vi "Enter_Temp_Press.vi"() -> ()   [LabVIEW 2013]
uses:
  Sub VIs/ADAM Controls/Ch_description_ADAM.ctl
  Sub VIs/ADAM Controls/Module_type_ADAM.ctl
  Sub VIs/ADAM Controls/Function_ADAM.ctl
  Sub VIs/ADAM Controls/Channel_State.ctl
  Sub VIs/ADAM Controls/Calib_type_ADAM.ctl
  Sub VIs/ADAM Controls/Address.ctl
  Anemometry/Anemometry Sub Vis/File/Setup_Filetype.ctl
  Sub VIs/ADAM Controls/Channel_names.ctl
  Anemometry/Anemometry Sub Vis/Controls/Preference_Mode.ctl
  Sub VIs/ADAM Controls/Update_scan_value.ctl
  Anemometry/Anemometry Sub Vis/Globals/Preference_global.vi
  Anemometry/Anemometry Sub Vis/Globals/Constants_global.vi
panel:
  in  "OK":bool
  out "Ch Description Array":T1[](array[typedef]) {"Duty" format="%.0b"; "D" format="%#_5g"; "C" format="%#_5g"; "B" format="%#_5g"; "A" format="%#_5g"}
  in  "mbars":dbl format="%#.1f"
  in  "Deg C":dbl format="%#.1f"
  in  "type specifier VI Refnum (for type only)":refnum<vi>
  out "Preference file":path
  in  "Server Comms":T7(ring)
  in  "Browse for Atmos Press":bool
  in  "Browse for Temp Ch":bool
  in  "Flow Pressure (Absolute) (mbars)":string="Froude:NPL:Atmos_Press"
  in  "Flow Temperature (deg C)":string="EnFlo Tun:Inlet Heater:Av Temp"
  # "DATA SOURCE"
  # "CURRENT VALUES"
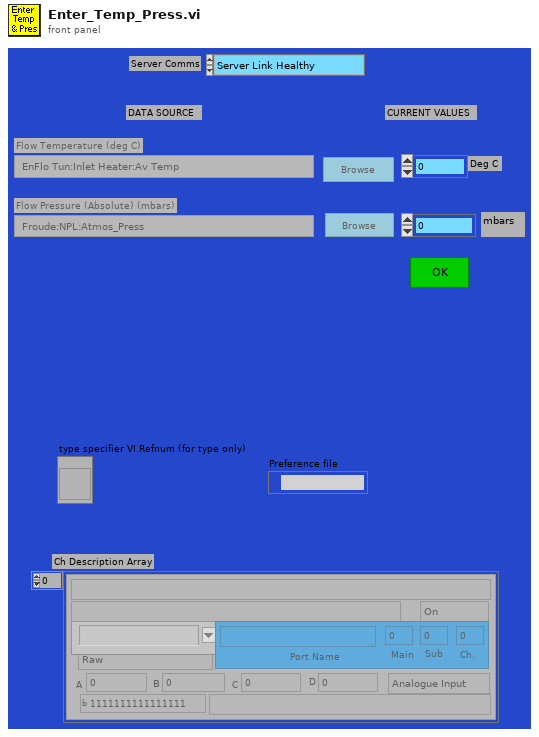
[diagram p1: front panel]
types:
  T1 = typedef "Ch_description_ADAM.ctl" = cluster{"Ch Name":string, "Type":T2, "Function":T3, "Ch State":T4, "Calibration type":T5, "A":dbl, "B":dbl, "C":dbl, "D":dbl, "Comments":string, "Address":T6, "String":string, "Duty":u16}
  T2 = typedef "Module_type_ADAM.ctl" = string
  T3 = typedef "Function_ADAM.ctl" = enum16{"Analogue Input", "Digital Input", "Event counter", "Event rate", "Analogue Output", "Digital Output", "Relay Output"}
  T4 = typedef "Channel_State.ctl" = enum16{"On", "Off", "Always On", "Always Off"}
  T5 = typedef "Calib_type_ADAM.ctl" = enum16{"Raw", "Bx + A", "Cx^2 + Bx + A", "Dx^3 + Cx^2 + Bx + A", "In Band", "Hi-Tec Q", "Hi-Tec M_dot", "Text"}
  T6 = typedef "Address.ctl" = cluster{"Main":i32, "Ch.":i32, "Sub":i32, "Port Name":string}
  T7 = enum16{"Server Link Healthy", "Do Not Link To Server"}
  T8 = typedef "Setup_Filetype.ctl" = enum16{"Measurement Setups", "Calibration Setups", "General", "Results File Plotter Setups", "Speed Calib Tweaks"}
  T9 = typedef "Channel_names.ctl" = enum16{"Active Only", "Active + Off", "All Channels"}
  T10 = enum16{"Zero or one", "One", "Zero or more", "One or more"}
  T11 = typedef "Preference_Mode.ctl" = enum16{"Load Preferences from file", "Save Preferences to file", "Load, Edit then Save"}
  T12 = typedef "Server_Comms.ctl" = enum16{"Server Link Healthy", "Do Not Link To Server"}
  T13 = typedef "Update_scan_value.ctl" = cluster{"Channel Name":string, "New Value":dbl}
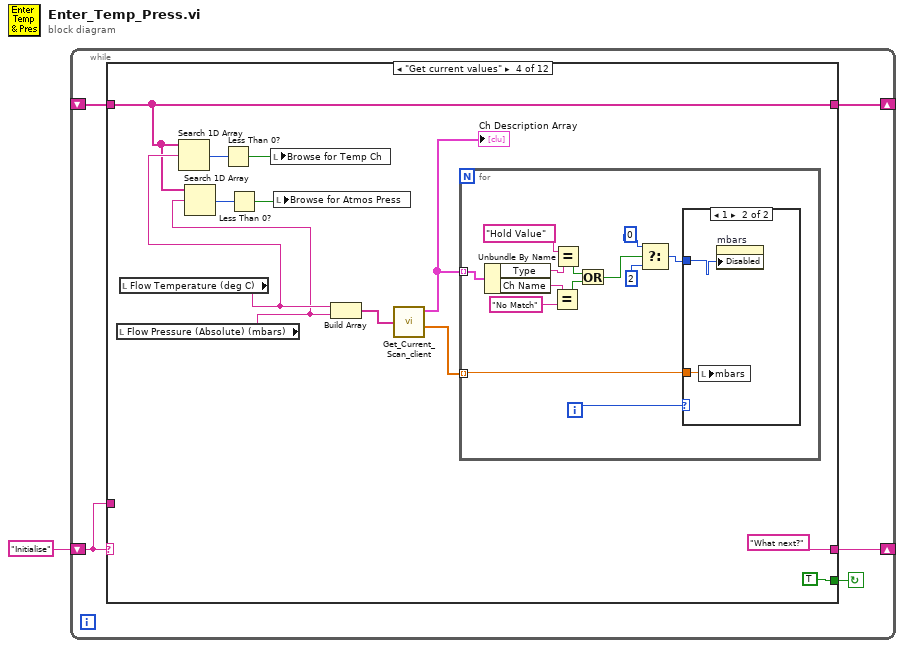
[diagram p0: block diagram]
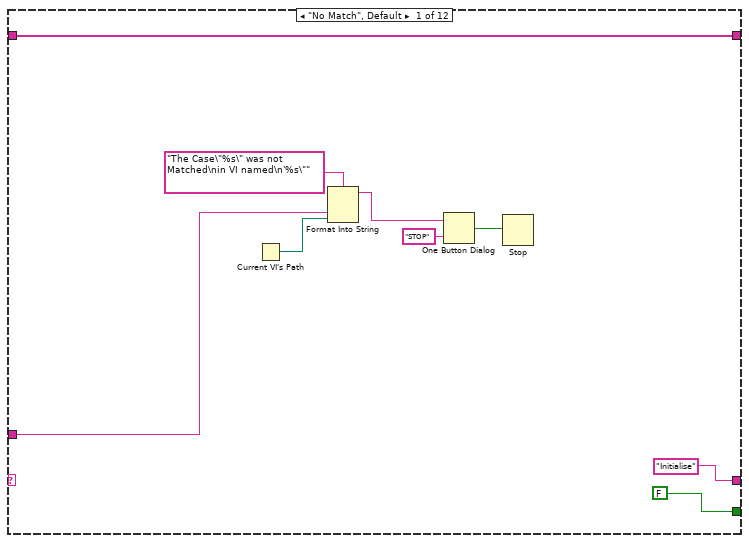
[diagram p2: hidden frame]
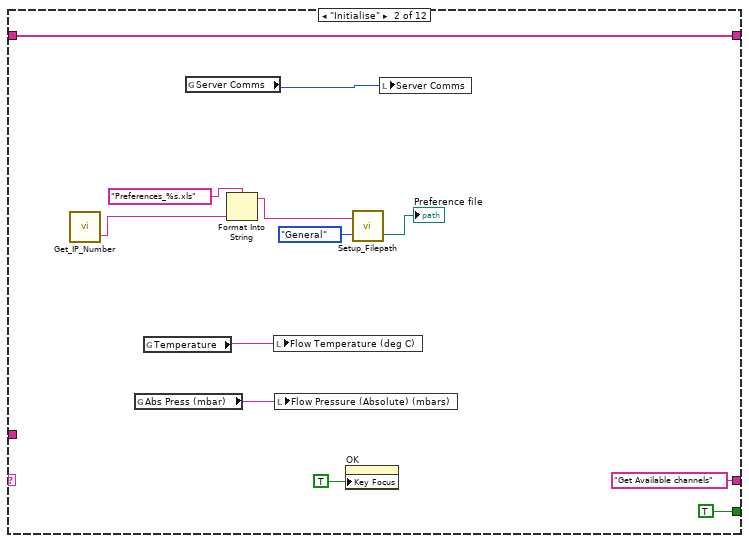
[diagram p3: hidden frame]
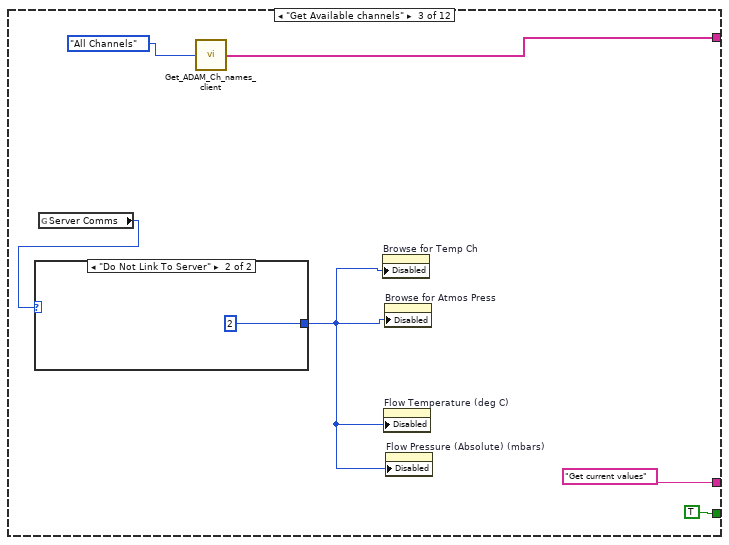
[diagram p4: hidden frame]
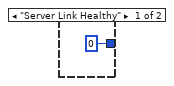
[diagram p5: hidden frame]
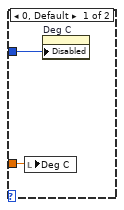
[diagram p6: hidden frame]
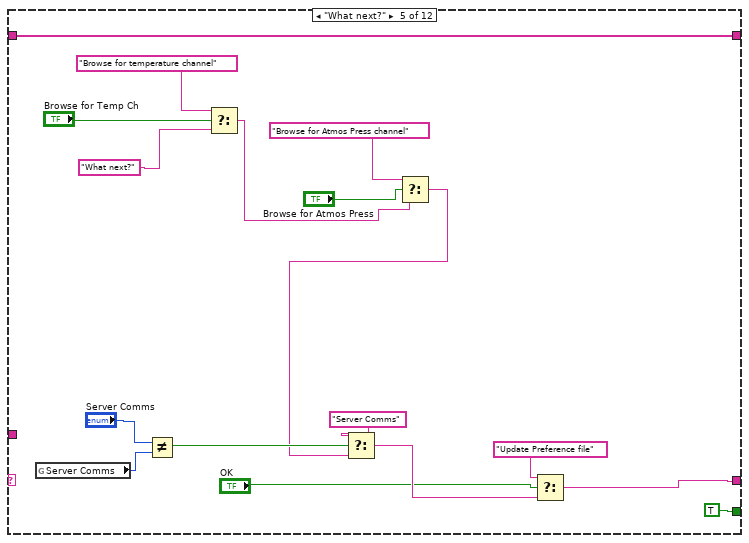
[diagram p7: hidden frame]
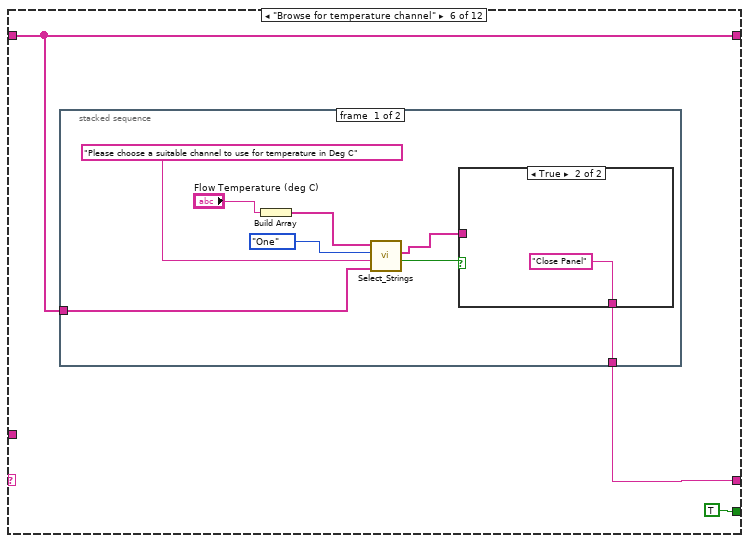
[diagram p8: hidden frame]
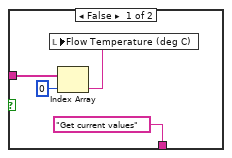
[diagram p9: hidden frame]
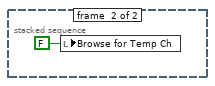
[diagram p10: hidden frame]
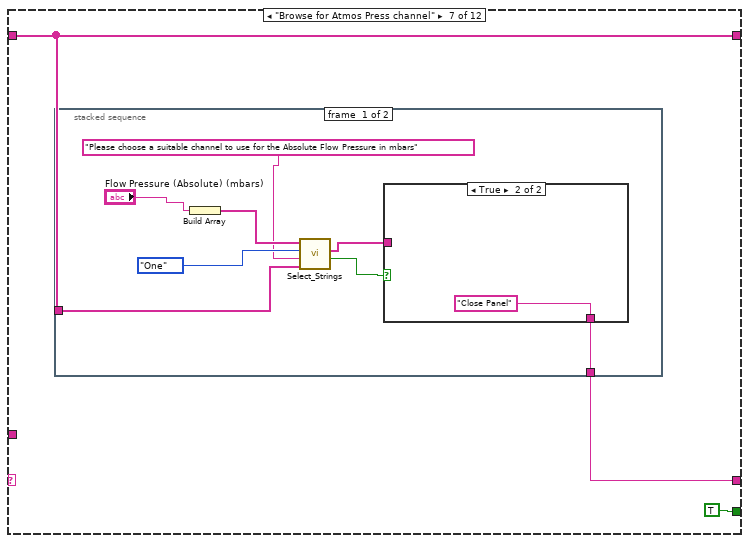
[diagram p11: hidden frame]
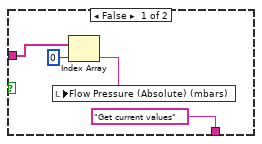
[diagram p12: hidden frame]
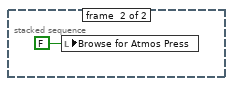
[diagram p13: hidden frame]
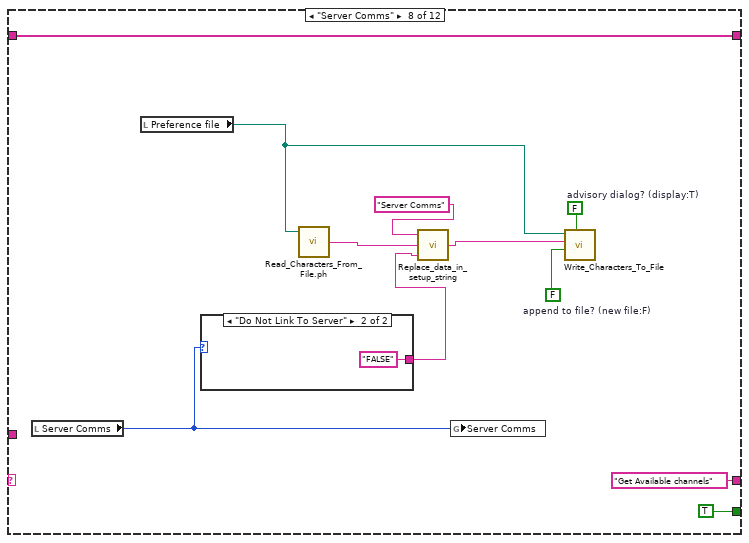
[diagram p14: hidden frame]
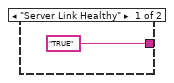
[diagram p15: hidden frame]
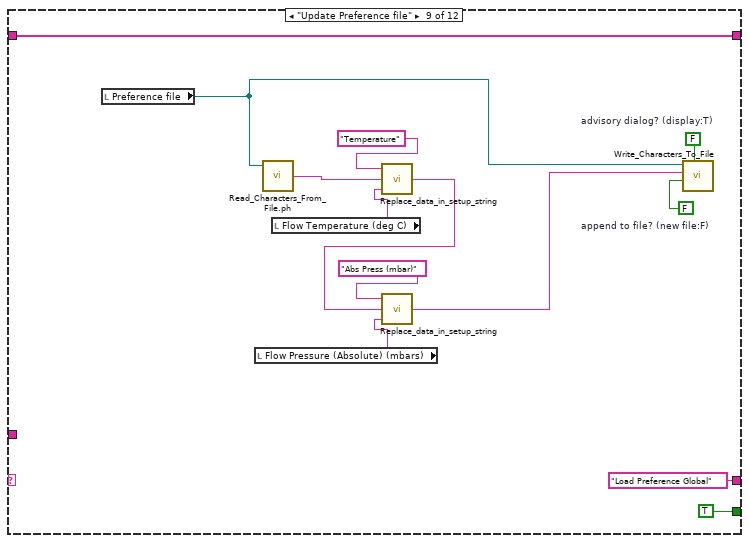
[diagram p16: hidden frame]
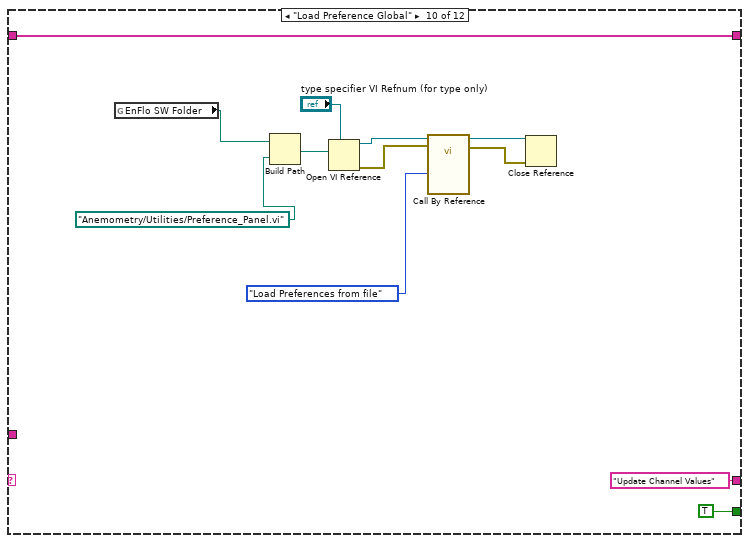
[diagram p17: hidden frame]
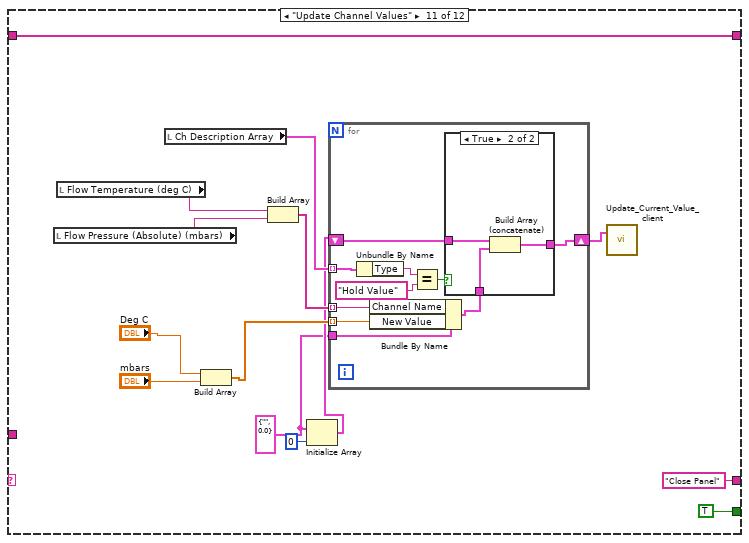
[diagram p18: hidden frame]
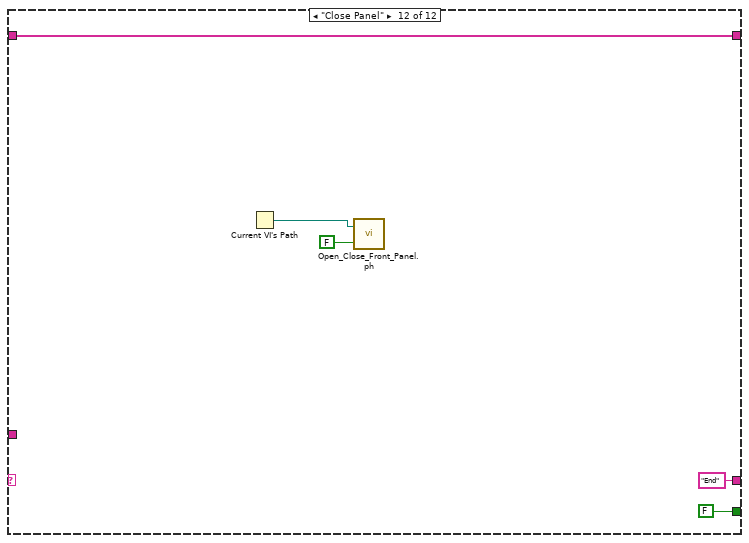
[diagram p20: hidden frame]
diagram:
  n1 = while {
    shift-left: "Initialise" -> [w4]
    shift-right: [w5] -> _
    shift-right: [w3] -> _
    shift-left: _ -> [w2]
    stop <- w6 continue-if-true
    n2 = case shown="\"Get current values\"" w4 {
      tunnel: [FALSE TRUE TRUE TRUE TRUE TRUE TRUE TRUE TRUE TRUE TRUE FALSE] -> w6
      tunnel: ["Initialise" "Get Available channels" "Get current values" "What next?" w78 w82 w99 "Get Available channels" "Load Preference Global" "Update Channel Values" "Close Panel" "End"] -> w5
      tunnel: w4 -> [w10 _ _ _ _ _ _ _ _ _ _ _]
      tunnel: [w7 w26 w30 w37 w75 w83 w100 w124 w139 w151 w165 w184] -> w3
      tunnel: w2 -> [w7 w26 _ w37 w75 w83 w100 w124 w139 w151 w165 w184]
      frame "No Match", Default {
        n3 = Current VI's Path() -> (path=w9:path)
        n4 = Format Into String(format string="The Case\"%s\" was not Matched\nin VI named\n'%s\"" ("Format String"), w10, w9) -> (resulting string=w13:string)  [unwired: 2 in, 1 out]
        n5 = One Button Dialog(message=w13, button name ("OK")="STOP") -> (true=w11:bool)
        n6 = Stop(stop? (T)=w11) -> ()
      }
      frame "Initialise" {
        n7 = call "Get_IP_Number.vi"() -> ("Computer Name"=w17:string)  [unwired: 1 out]
        n8 = global read "Preference_global.vi" "Abs Press (mbar)"() -> (w23:string)
        n9 = global read "Preference_global.vi" "Temperature"() -> (w22:string)
        n10 = global read "Preference_global.vi" "Server Comms"() -> (w27:T12)
        n11 = Format Into String(format string="Preferences_%s.xls" ("name or relative path"), w17) -> (resulting string=w18:string)  [unwired: 2 in, 1 out]
        n12 = local write "Flow Temperature (deg C)"(w22) -> ()
        n13 = local write "Flow Pressure (Absolute) (mbars)"(w23) -> ()
        n14 = property on="OK" class="Bool"("Key Focus"=TRUE) -> ()  [unwired: 2 in, 2 out]
        n15 = call "Setup_Filepath.vi"("Setup File Type"=Setup_Filetype."General", "Filename in"=w18) -> ("Filename Out"=→"Preference file":path)  [unwired: 1 out]
        n16 = local write "Server Comms"(w27) -> ()
      }
      frame "Get Available channels" {
        n17 = global read "Preference_global.vi" "Server Comms"() -> (w29:T12)
        n18 = case shown="\"Do Not Link To Server\"" w29 {
          tunnel: [u8 0 ("Disabled") u8 2 ("Disabled")] -> w28
          frame "Server Link Healthy" {
          }
          frame "Do Not Link To Server" {
          }
        }
        n19 = call "Get_ADAM_Ch_names_client.vi"("Channel names set"=Channel_names."All Channels") -> ("Ch names"=w30:string[])
        n20 = property on="Browse for Temp Ch" class="Bool (strict)"("Disabled"=w28) -> ()  [unwired: 2 in, 2 out]
        n21 = property on="Flow Temperature (deg C)" class="Str"("Disabled"=w28) -> ()  [unwired: 2 in, 2 out]
        n22 = property on="Browse for Atmos Press" class="Bool (strict)"("Disabled"=w28) -> ()  [unwired: 2 in, 2 out]
        n23 = property on="Flow Pressure (Absolute) (mbars)" class="Str"("Disabled"=w28) -> ()  [unwired: 2 in, 2 out]
      }
      frame "Get current values" {
        n24 = local read "Flow Pressure (Absolute) (mbars)"() -> (w36:string)
        n25 = local read "Flow Temperature (deg C)"() -> (w42:string)
        n26 = Search 1D Array(1D array=w37, element=w42) -> (index of element=w41:i32)  [unwired: 1 out]
        n27 = Search 1D Array(1D array=w37, element=w36) -> (index of element=w40:i32)  [unwired: 1 out]
        n28 = Less Than 0?(x=w41) -> (x < 0?=w39:bool)
        n29 = Less Than 0?(x=w40) -> (x < 0?=w38:bool)
        n30 = local write "Browse for Temp Ch"(w39) -> ()
        n31 = local write "Browse for Atmos Press"(w38) -> ()
        n32 = Build Array(w42, w36) -> (w45:string[])
        n33 = call "Get_Current_Scan_client.vi"("ADAM Ch Names"=w45) -> ("Ch Description Array"=w43:T1[], "Numerical Values"=w44:dbl[])  [unwired: 1 in, 1 out]
        "Ch Description Array" <- w43
        n34 = for {
          tunnel: w44 -> [w51] mode=indexing
          tunnel: w43 -> [w48] mode=indexing
          i -> [w60]
          n35 = Unbundle By Name(w48) -> ("Type"=w50:T2, "Ch Name"=w49:string)
          n36 = Equal?(x=w49, y="No Match") -> (x = y?=w54:bool)
          n37 = Equal?(x=T2 "Hold Value" ("Type"), y=w50) -> (x = y?=w53:bool)
          n38 = Or(x=w53, y=w54) -> (x .or. y?=w52:bool)
          n39 = Select(t=u8 0 ("Disabled"), s=w52, f=u8 2 ("Disabled")) -> (s? t:f=w56:u8)
          n40 = case shown="1" w60 {
            tunnel: w51 -> [w62 w64]
            tunnel: w56 -> [w61 w63]
            frame 0, Default {
              n41 = local write "Deg C"(w62) -> ()
              n42 = property on="Deg C" class="DigNum (strict)"("Disabled"=w61) -> ()  [unwired: 2 in, 2 out]
            }
            frame 1 {
              n43 = local write "mbars"(w64) -> ()
              n44 = property on="mbars" class="DigNum (strict)"("Disabled"=w63) -> ()  [unwired: 2 in, 2 out]
            }
          }
        }
      }
      frame "What next?" {
        n45 = global read "Preference_global.vi" "Server Comms"() -> (w69:T12)
        n46 = Not Equal?(x="Server Comms", y=w69) -> (x != y?=w67:bool)
        n47 = Select(t="Browse for temperature channel", s="Browse for Temp Ch", f="What next?") -> (s? t:f=w72:string)
        n48 = Select(t="Browse for Atmos Press channel", s="Browse for Atmos Press", f=w72) -> (s? t:f=w65:string)
        n49 = Select(t="Server Comms", s=w67, f=w65) -> (s? t:f=w71:string)
        n50 = Select(t="Update Preference file", s="OK", f=w71) -> (s? t:f=w78:string)
      }
      frame "Browse for temperature channel" {
        n51 = stacked-sequence {
          tunnel: w83 -> [w90 _]
          tunnel: [w85 _] -> w82
          frame #0 {
            n52 = Build Array("Flow Temperature (deg C)") -> (w92:string[])
            n53 = call "Select_Strings.vi"("Available Ch names"=w90, "Message"="Please choose a suitable channel to use for temperature in Deg C", "Selector mode"=T10."One", "Desired Ch names (in)"=w92) -> ("Cancel"=w86:bool, "Selected Channel Names"=w89:string[])  [unwired: 3 out]
            n54 = case shown="True" w86 {
              tunnel: w89 -> [w96 _]
              tunnel: ["Get current values" "Close Panel"] -> w85
              frame False {
                n55 = Index Array(array=w96, index=0) -> (element=w94:string)
                n56 = local write "Flow Temperature (deg C)"(w94) -> ()
              }
              frame True {
              }
            }
          }
          frame #1 {
            n57 = local write "Browse for Temp Ch"(FALSE ("Browse for Temp Ch")) -> ()
          }
        }
      }
      frame "Browse for Atmos Press channel" {
        n58 = stacked-sequence {
          tunnel: w100 -> [w107 _]
          tunnel: [w102 _] -> w99
          frame #0 {
            n59 = Build Array("Flow Pressure (Absolute) (mbars)") -> (w109:string[])
            n60 = call "Select_Strings.vi"("Available Ch names"=w107, "Message"="Please choose a suitable channel to use for the Absolute Flow Pressure in mbars", "Selector mode"=T10."One", "Desired Ch names (in)"=w109) -> ("Cancel"=w103:bool, "Selected Channel Names"=w106:string[])  [unwired: 3 out]
            n61 = case shown="True" w103 {
              tunnel: w106 -> [w113 _]
              tunnel: ["Get current values" "Close Panel"] -> w102
              frame False {
                n62 = Index Array(array=w113, index=0) -> (element=w111:string)
                n63 = local write "Flow Pressure (Absolute) (mbars)"(w111) -> ()
              }
              frame True {
              }
            }
          }
          frame #1 {
            n64 = local write "Browse for Atmos Press"(FALSE ("Browse for Atmos Press")) -> ()
          }
        }
      }
      frame "Server Comms" {
        w123 = FALSE  # append to file? (new file:F)
        w122 = FALSE  # advisory dialog? (display:T)
        n65 = local read "Server Comms"() -> (w117:T7)
        n66 = local read "Preference file"() -> (w119:path)
        n67 = case shown="\"Do Not Link To Server\"" w117 {
          tunnel: ["TRUE" "FALSE"] -> w116
          frame "Server Link Healthy" {
          }
          frame "Do Not Link To Server" {
          }
        }
        n68 = call "Read_Characters_From_File.ph.vi"("file path (dialog if empty)"=w119) -> ("character string"=w121:string)  [unwired: 1 in, 7 out]
        n69 = call "Replace_data_in_setup_string.vi"("New data string"=w116, "Input string"=w121, "Variable name"="Server Comms") -> ("Appended string"=w120:string)
        n70 = global write "Preference_global.vi" "Server Comms"(w117) -> ()
        n71 = call "Write_Characters_To_File.vi"("file path (dialog if empty)"=w119, "advisory dialog? (display:T)"=w122, "character string"=w120, "append to file? (new file:F)"=w123) -> ()  [unwired: 1 in, 4 out]
      }
      frame "Update Preference file" {
        w138 = FALSE  # append to file? (new file:F)
        w137 = FALSE  # advisory dialog? (display:T)
        n72 = local read "Preference file"() -> (w135:path)
        n73 = local read "Flow Pressure (Absolute) (mbars)"() -> (w132:string)
        n74 = call "Read_Characters_From_File.ph.vi"("file path (dialog if empty)"=w135) -> ("character string"=w136:string)  [unwired: 1 in, 7 out]
        n75 = local read "Flow Temperature (deg C)"() -> (w133:string)
        n76 = call "Replace_data_in_setup_string.vi"("New data string"=w133, "Input string"=w136, "Variable name"="Temperature") -> ("Appended string"=w130:string)
        n77 = call "Replace_data_in_setup_string.vi"("New data string"=w132, "Input string"=w130, "Variable name"="Abs Press (mbar)") -> ("Appended string"=w129:string)
        n78 = call "Write_Characters_To_File.vi"("file path (dialog if empty)"=w135, "advisory dialog? (display:T)"=w137, "character string"=w129, "append to file? (new file:F)"=w138) -> ()  [unwired: 1 in, 4 out]
      }
      frame "Load Preference Global" {
        n79 = global read "Constants_global.vi" "EnFlo SW Folder"() -> (w144:path)
        n80 = Build Path(base path=w144, name or relative path=path "Anemometry/Utilities/Preference_Panel.vi") -> (appended path=w146:path)
        n81 = Open VI Reference(type specifier VI Refnum (for type only)="type specifier VI Refnum (for type only)", vi path=w146) -> (vi reference=w147:refnum<vi>, error out=w148:errorcluster)  [unwired: 1 in, 3 out]
        n82 = call-by-ref "?"(reference=w147, error in=w148, "Mode"=Preference_Mode."Load Preferences from file") -> (reference out=w149:refnum<vi>, error out=w150:errorcluster)
        n83 = Close Reference(reference=w149, error in (no error)=w150) -> ()  [unwired: 1 out]
      }
      frame "Update Channel Values" {
        w155 = T13 {"Channel Name"="", "New Value"=0.0} ("Update Scan Value Cluster")
        n84 = local read "Flow Pressure (Absolute) (mbars)"() -> (w162:string)
        n85 = local read "Flow Temperature (deg C)"() -> (w161:string)
        n86 = local read "Ch Description Array"() -> (w158:T1[])
        n87 = Build Array("Deg C", "mbars") -> (w159:dbl[])
        n88 = Build Array(w161, w162) -> (w160:string[])
        n89 = Initialize Array(w155, 0 ("dimension size")) -> (w156:T13[])
        n90 = for {
          shift-right: [w169] -> w154
          shift-left: w156 -> [w171]
          tunnel: w160 -> [w177] mode=indexing
          tunnel: w159 -> [w176] mode=indexing
          tunnel: w158 -> [w175] mode=indexing
          tunnel: w155 -> [w168]
          n91 = Unbundle By Name(w175) -> ("Type"=w173:T2)
          n92 = Bundle By Name(cluster=w168, "Channel Name"=w177, "New Value"=w176) -> (w170:T13)
          n93 = Equal?(x=w173, y=T2 "Hold Value" ("Type")) -> (x = y?=w172:bool)
          n94 = case shown="True" w172 {
            tunnel: w171 -> [w178 w181]
            tunnel: w170 -> [_ w180]
            tunnel: [w178 w179] -> w169
            frame False {
            }
            frame True {
              n95 = Build Array (concatenate)(w181, w180) -> (w179:T13[])
            }
          }
        }
        n96 = call "Update_Current_Value_client.vi"("Update array in"=w154) -> ()  [unwired: 1 in]
      }
      frame "Close Panel" {
        n97 = Current VI's Path() -> (path=w183:path)
        n98 = call "Open_Close_Front_Panel.ph.vi"("Front Panel Window:Open"=FALSE, "VI path"=w183) -> ()  [unwired: 2 out]
      }
    }
  }
